vi "Eval y=f(x) Prep2 .vi"(2 "epsilon":dbl format="%.2f", 3 "Parsed Formula":cluster{"Table":i32[][], "Y Values":dbl[]} {"Y Values" format="%.2f"}, 4 "random summand":dbl format="%.2f", 5 "points II in":dbl[](array[numeric]) format="%.2f", 6 "points I in":dbl[](array[numeric]) format="%.2f", 7 "points in":dbl[](array[numeric]) format="%.2f") -> (0 "points I out":dbl[](array[numeric]) format="%.2f", 1 "points out":dbl[](array[numeric]) format="%.2f")   [LabVIEW 2017, in "NI_Gmath.lvlib"]
uses:
  NI_Gmath.lvlib
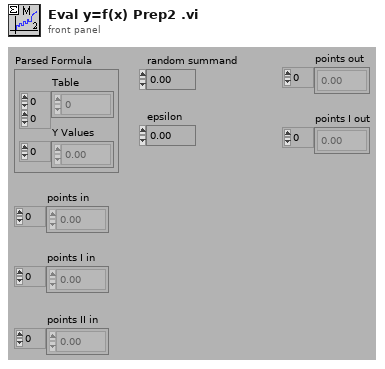
[diagram p1: front panel]
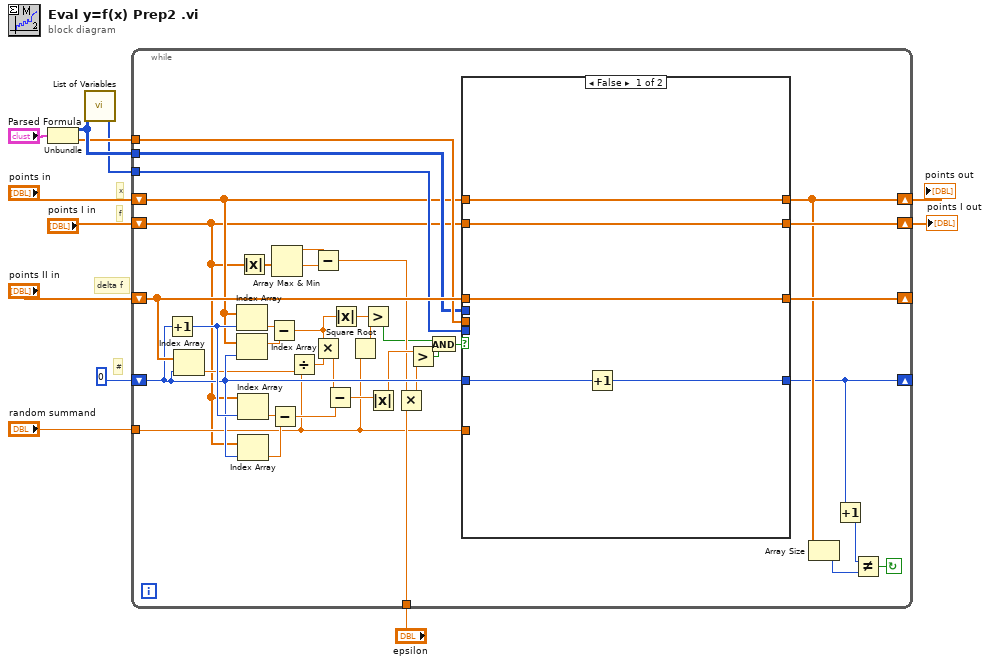
[diagram p0: block diagram]
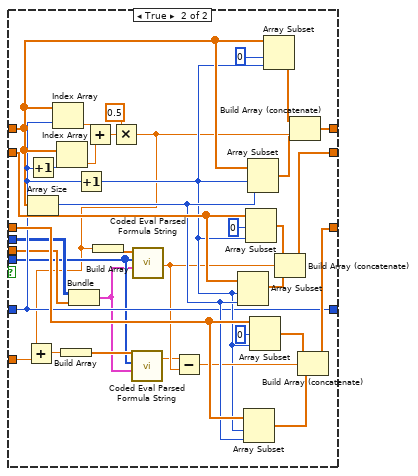
[diagram p2: hidden frame]
diagram:
  # "#"
  # "delta f"
  # "f"
  # "x"
  n1 = Unbundle("Parsed Formula") -> ("Table"=w12:i32[][], "Y Values"=w11:dbl[])
  n2 = call "List of Variables.vi"("Table"=w12) -> ("List of variables"=w4:i32[])
  n3 = while {
    tunnel: w4 -> [w41]
    tunnel: w12 -> [w42]
    tunnel: w11 -> [w43]
    tunnel: "epsilon" -> [w33]
    tunnel: "random summand" -> [w18]
    shift-left: 0 -> [w39]
    shift-right: [w45] -> _
    shift-left: "points II in" -> [w46]
    shift-right: [w49] -> _
    shift-left: "points I in" -> [w13]
    shift-right: [w50] -> w8
    shift-left: "points in" -> [w14]
    shift-right: [w48] -> w7
    stop <- w47 continue-if-true
    n4 = Increment(x=w39) -> (x+1=w40:i32)
    n5 = Index Array(array=w46, index=w39) -> (element=w26:dbl)
    n6 = Index Array(array=w14, index=w40) -> (element=w30:dbl)
    n7 = Index Array(array=w14, index=w39) -> (element=w29:dbl)
    n8 = Index Array(array=w13, index=w40) -> (element=w28:dbl)
    n9 = Index Array(array=w13, index=w39) -> (element=w27:dbl)
    n10 = Absolute Value(x=w13) -> (abs(x)=w34:dbl[])
    n11 = Subtract(x=w30, y=w29) -> (x-y=w20:dbl)
    n12 = Subtract(x=w28, y=w27) -> (x-y=w36:dbl)
    n13 = Array Max & Min(array=w34) -> (max value=w25:dbl, min value=w24:dbl)  [unwired: 2 out]
    n14 = Divide(x=w26, y=w18) -> (x/y=w38:dbl)
    n15 = Subtract(x=w25, y=w24) -> (x-y=w23:dbl)
    n16 = Multiply(x=w20, y=w38) -> (x*y=w37:dbl)
    n17 = Subtract(x=w37, y=w36) -> (x-y=w35:dbl)
    n18 = Absolute Value(x=w20) -> (abs(x)=w19:dbl)
    n19 = Square Root(x=w18) -> (sqrt(x)=w15:dbl)
    n20 = Greater?(x=w19, y=w15) -> (0:w17:bool)
    n21 = Absolute Value(x=w35) -> (abs(x)=w32:dbl)
    n22 = Multiply(x=w23, y=w33) -> (x*y=w31:dbl)
    n23 = Greater?(x=w32, y=w31) -> (0:w21:bool)
    n24 = And(x=w17, y=w21) -> (x .and. y?=w16:bool)
    n25 = case shown="False" w16 {
      tunnel: w39 -> [w52 w66]
      tunnel: w14 -> [w55 w81]
      tunnel: [w55 w83] -> w48
      tunnel: w13 -> [w54 w79]
      tunnel: [w54 w69] -> w50
      tunnel: w46 -> [w53 w75]
      tunnel: [w53 w68] -> w49
      tunnel: w18 -> [_ w76]
      tunnel: [w51 w66] -> w45
      tunnel: w43 -> [_ w61]
      tunnel: w42 -> [_ w62]
      tunnel: w41 -> [_ w58]
      frame False {
        n26 = Increment(x=w52) -> (x+1=w51:i32)
      }
      frame True {
        n27 = Increment(x=w66) -> (x+1=w90:i32)
        n28 = Array Size(array=w81) -> (size(s)=w71:i32)
        n29 = Index Array(array=w81, index=w66) -> (element=w89:dbl)
        n30 = Index Array(array=w81, index=w90) -> (element=w88:dbl)
        n31 = Bundle("Table"=w62, "Y Values"=w61) -> (w57:cluster{"Table":i32[][], "Y Values":dbl[]})  [unwired: 1 in]
        n32 = Increment(x=w66) -> (x+1=w67:i32)
        n33 = Add(x=w89, y=w88) -> (x+y=w87:dbl)
        n34 = Multiply(x=0.5, y=w87) -> (x*y=w56:dbl)
        n35 = Add(x=w56, y=w76) -> (x+y=w64:dbl)
        n36 = Build Array(w64) -> (w59:dbl[])
        n37 = Build Array(w56) -> (w60:dbl[])
        n38 = call "Coded Eval Parsed Formula String.vi"("Parsed Formula"=w57, "Variables"=w58, "X Values"=w59) -> ("y value"=w63:dbl)  [unwired: 1 in, 1 out]
        n39 = call "Coded Eval Parsed Formula String.vi"("Parsed Formula"=w57, "Variables"=w58, "X Values"=w60) -> ("y value"=w65:dbl)  [unwired: 1 in, 1 out]
        n40 = Subtract(x=w63, y=w65) -> (x-y=w70:dbl)
        n41 = Array Subset(array=w79, index=w67, length=w71) -> (w77:dbl[])
        n42 = Array Subset(array=w75, index=w67, length=w71) -> (w72:dbl[])
        n43 = Array Subset(array=w79, index=0, length=w67) -> (w78:dbl[])
        n44 = Array Subset(array=w81, index=w67, length=w71) -> (w84:dbl[])
        n45 = Array Subset(array=w75, index=0, length=w67) -> (w73:dbl[])
        n46 = Array Subset(array=w81, index=0, length=w67) -> (w85:dbl[])
        n47 = Build Array (concatenate)(w78, w65, w77) -> (w69:dbl[])
        n48 = Build Array (concatenate)(w85, w56, w84) -> (w83:dbl[])
        n49 = Build Array (concatenate)(w73, w70, w72) -> (w68:dbl[])
      }
    }
    n50 = Array Size(array=w48) -> (size(s)=w22:i32)
    n51 = Increment(x=w45) -> (x+1=w44:i32)
    n52 = Not Equal?(x=w44, y=w22) -> (x != y?=w47:bool)
  }
  "points I out" <- w8
  "points out" <- w7
